vi "Add LV Passwords.vi"(8 "error in (no error)":errorcluster) -> (0 "error out":errorcluster)   [LabVIEW 2020]
panel:
  in  "Passwords Array":string[](array[string])=[".labviewrc", "4xtddatamunge", "73LV6i49EVAL18", "AxisOfEval", "CanadianContent", "Everest Trek", "Express rocks, baby!", "GotZoomZoom?", "HoldYourPeas", "JackBlack", "NewToMe", "RatzFatz", "SuperSecretSimulation", "TDIter", "as-seen-on.tv", "bergamot", "birdie", "casa de luz", "changeslost", "depechemode", "diagramarama", "echoskye", "estoy listo, jefe!", "fabulous manzier bros", "finger wech", "fiziks", "formica21", "g-sizer", "gURLpower", "gandalf_vs_merlin_43babelfish_would_be_funny", "geewiz", "ghostinabikini", "goingcommando", "goop rules", "gregr", "habitat_shelter_327_(YodaHut)", "hepsi senin mi", "ic.what.rtcs", "incipient", "it_all_starts_8468_here", "jabberwocky", "labv1ew", "like_a_5969_rolling_stone", "linus_10299_blanket", "littlegreenman", "lookingglass", "lvfpga2003", "lvfpga2004rio", "lvfpga2004", "maple leaf", "mcqueen", "mytwocents", "nifind", "round mango", "rt.magic 42", "sassifrass", "scriptonly", "somethingisrottenindenmark", "stupid is as stupid does", "stupidisasstupiddoes", "superdupertl", "surfin", "takethebluepill", "yushiscope", "zilker_51797_umlauf", "CandyMountain4U"]
  # "Adding passwords...please wait"
  # "This VI contains the known passwords of all the VI-based\ndialogs in LabVIEW.  If you receive an error from the dialog\npopulator that a VI has an incorrect password, look at the\npasswords.txt file in Perforce and add the new password\nto this list.  Don't forget to \"Make Current Value Default\" before\nsaving this VI."
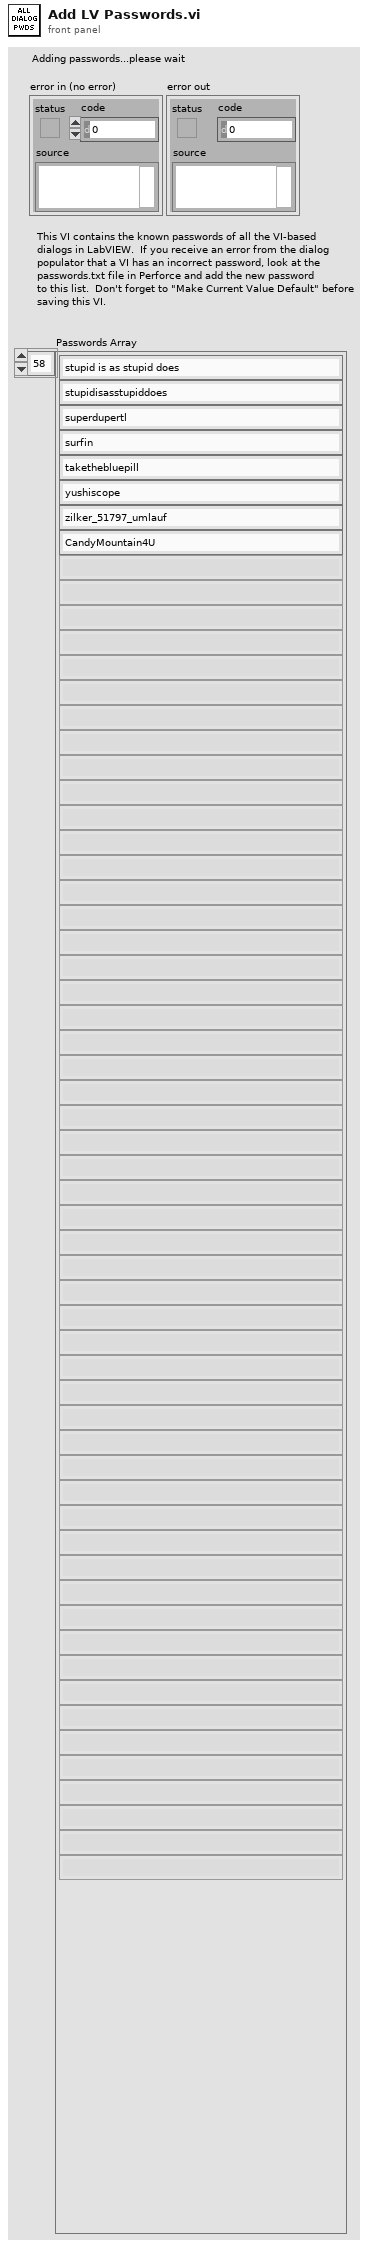
[diagram p1: front panel]
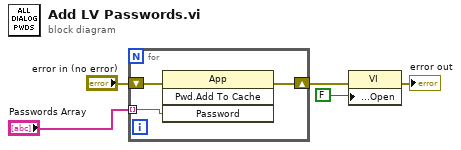
[diagram p0: block diagram]
diagram:
  n1 = for {
    tunnel: "Passwords Array" -> [w7] mode=indexing
    shift-right: [w6] -> w4
    shift-left: "error in (no error)" -> [w8]
    n2 = invoke class="App" method="Pwd.Add To Cache"(error in=w8, "Password"=w7) -> (error out=w6:errorcluster)  [unwired: 2 in, 3 out]
  }
  n3 = property class="VI"(error in=w4, "Front Panel Window:Open"=FALSE) -> (error out=→"error out":errorcluster)  [unwired: 1 in, 1 out]
